vi "Verify Variants.vi"(0 "Expected Values":T1={"Boolean"=TRUE, "Numeric"=4, "String"="hello", "Boolean Array"=[TRUE, FALSE, TRUE, FALSE], "String Array"=["str1", "str2", "str3"], "Numeric Array"=[1.0, 2.0, 3.0]} {"Numeric Array" format="%0.2f"}, 5 "Boolean Variant":variant=variant(bool TRUE), 7 "Numeric Variant":variant=variant(dbl 4.0) caption="Numeric Variant Caption", 9 "String Variant":variant=variant(string "hello"), 11 "Boolean Array Variant":variant=variant(bool[] [TRUE, FALSE, TRUE, FALSE]), 12 "Numeric Array Variant":variant=variant(u8[] [1, 2, 3]), 13 "String Array Variant":variant=variant(string[] ["str1", "str2", "str3"])) -> (4 "All Values Are Equal":bool)   [LabVIEW 2012]
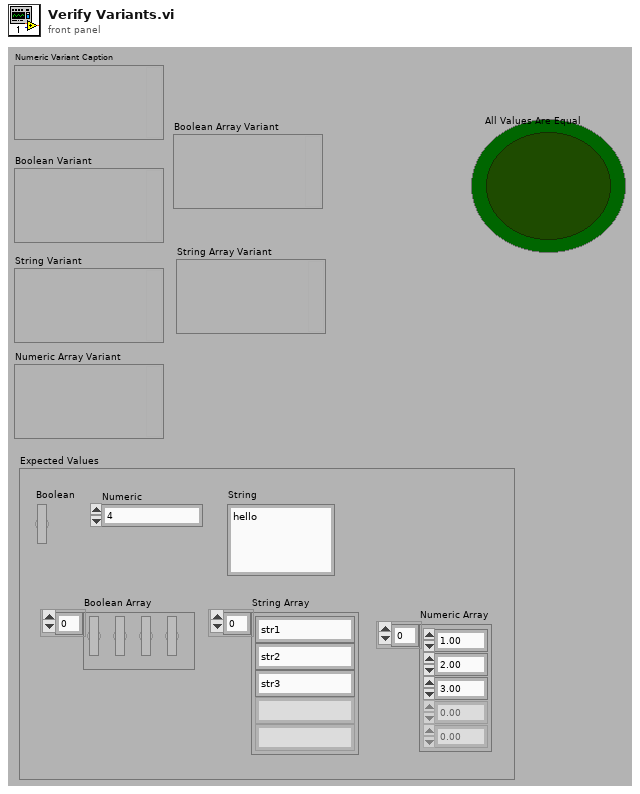
[diagram p1: front panel]
types:
  T1 = cluster{"Boolean":bool, "Numeric":u32, "String":string, "Boolean Array":bool[], "String Array":string[], "Numeric Array":dbl[]}
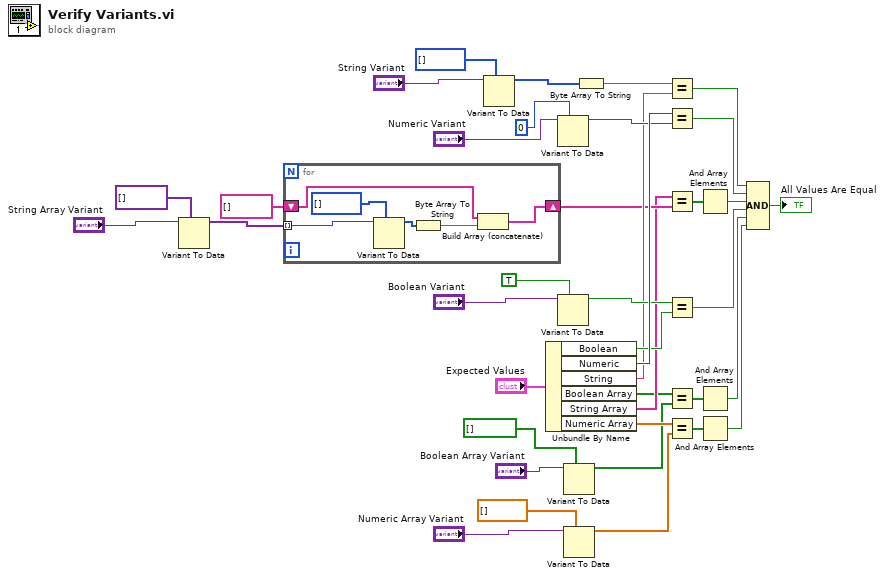
[diagram p0: block diagram]
diagram:
  n1 = Variant To Data(type=variant[] [], Variant="String Array Variant") -> (data=w16:variant[])  [unwired: 1 in, 1 out]
  n2 = for {
    tunnel: w16 -> [w44] mode=indexing
    shift-right: [w40] -> w14
    shift-left: string[] [] -> [w41]
    n3 = Variant To Data(type=u8[] [], Variant=w44) -> (data=w42:u8[])  [unwired: 1 in, 1 out]
    n4 = Byte Array To String(unsigned byte array=w42) -> (string=w39:string)
    n5 = Build Array (concatenate)(w41, w39) -> (w40:string[])
  }
  n6 = Variant To Data(type=u8[] [], Variant="String Variant") -> (data=w23:u8[])  [unwired: 1 in, 1 out]
  n7 = Unbundle By Name("Expected Values") -> ("Boolean"=w27:bool, "Numeric"=w30:u32, "String"=w25:string, "Boolean Array"=w12:bool[], "String Array"=w13:string[], "Numeric Array"=w19:dbl[])
  n8 = Variant To Data(type=u32 0, Variant="Numeric Variant") -> (data=w29:u32)  [unwired: 1 in, 1 out]
  n9 = Variant To Data(type=TRUE, Variant="Boolean Variant") -> (data=w26:bool)  [unwired: 1 in, 1 out]
  n10 = Variant To Data(type=bool[] [], Variant="Boolean Array Variant") -> (data=w11:bool[])  [unwired: 1 in, 1 out]
  n11 = Variant To Data(type=dbl[] [], Variant="Numeric Array Variant") -> (data=w20:dbl[])  [unwired: 1 in, 1 out]
  n12 = Byte Array To String(unsigned byte array=w23) -> (string=w22:string)
  n13 = Equal?(x=w22, y=w25) -> (x = y?=w7:bool)
  n14 = Equal?(x=w30, y=w29) -> (x = y?=w6:bool)
  n15 = Equal?(x=w13, y=w14) -> (x = y?=w8:bool[])
  n16 = Equal?(x=w26, y=w27) -> (x = y?=w4:bool)
  n17 = Equal?(x=w12, y=w11) -> (x = y?=w9:bool[])
  n18 = Equal?(x=w19, y=w20) -> (x = y?=w10:bool[])
  n19 = And Array Elements(Boolean array=w8) -> (logical AND=w5:bool)
  n20 = And Array Elements(Boolean array=w9) -> (logical AND=w3:bool)
  n21 = And Array Elements(Boolean array=w10) -> (logical AND=w2:bool)
  n22 = Compound Arithmetic op=AND(w7, w6, w5, w4, w3, w2) -> (→"All Values Are Equal":bool)
